vi "验证均匀分布.vi"() -> ()   [LabVIEW 2012]
uses:
  <vilib>/Analysis/NI_AALBase.lvlib
panel:
  out "方差":dbl
  out "期望值":dbl
  out "variance":dbl caption="方差" format="%0.8f"
  out "mean":dbl caption="均值" format="%0.8f"
  out "MSE":dbl format="%0.8f"
  out "Mean":dbl format="%#_8f"
  in  "Num":i32
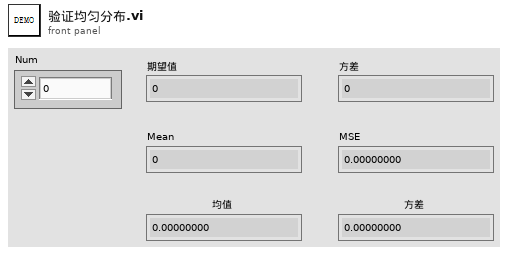
[diagram p1: front panel]
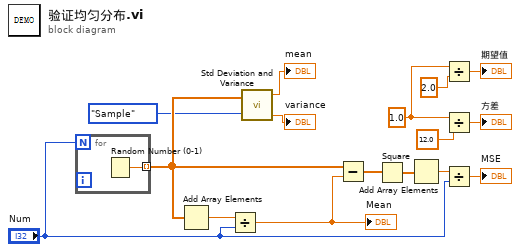
[diagram p0: block diagram]
diagram:
  w3 = 1.0
  n1 = for {
    N: "Num" -> [_]
    tunnel: [w17] -> w9 mode=indexing
    n2 = Random Number (0-1)() -> (number: 0 to 1=w17:dbl)
  }
  n3 = Add Array Elements(numeric array=w9) -> (sum=w16:dbl)
  n4 = Divide(x=w16, y="Num") -> (x/y=w15:dbl)
  "Mean" <- w15
  n5 = call <vilib>:"Std Deviation and Variance.vi"("X"=w9, "Weighting (Sample)"=enum16{"Sample", "Population"}."Sample") -> ("mean"=→"mean":dbl, "variance"=→"variance":dbl)  [unwired: 1 out]
  n6 = Subtract(x=w9, y=w15) -> (x-y=w14:dbl[])
  n7 = Square(x=w14) -> (x^2=w13:dbl[])
  n8 = Add Array Elements(numeric array=w13) -> (sum=w12:dbl)
  n9 = Divide(x=w3, y=2.0) -> (x/y=→"期望值":dbl)
  n10 = Divide(x=w3, y=12.0) -> (x/y=→"方差":dbl)
  n11 = Divide(x=w12, y="Num") -> (x/y=→"MSE":dbl)
